vi "2_VisualizeModulePositioning.vi"(0 "Session in":T1, 1 "Calibrated positions of fiducials [mm]":dbl[][](array[numeric])=[[-675.4228165149058, -196.82430550413875, -11.55], [-579.8428201474238, -196.8506568257386, -11.55], [-579.816468825824, -101.27066045825673, -11.55], [-675.3964651933059, -101.24430913665685, -11.55], [-577.422820239396, -196.8513240176017, -11.55], [-481.84282387191405, -196.87767533920157, -11.55], [-481.8164725503142, -101.29767897171968, -11.55], [-577.396468917796, -101.2713276501198, -11.55], [-479.42282396388623, -196.87834253106465, -11.55], [-383.8428275964043, -196.90469385266454, -11.55], [-383.81647627480436, -101.32469748518264, -11.55], [-479.3964726422863, -101.29834616358275, -11.55], [-381.42282768837646, -196.90536104452758, -11.55], [-285.8428313208945, -196.93171236612747, -11.55], [-285.8164799992946, -101.35171599864559, -11.55], [-381.39647636677654, -101.3253646770457, -11.55], [-283.4228314128667, -196.93237955799054, -11.55], [-187.84283504538473, -196.95873087959043, -11.55], [-187.8164837237848, -101.37873451210854, -11.55], [-283.39648009126677, -101.35238319050865, -11.55], [-185.42283513735697, -196.9593980714535, -11.55], [-89.84283876987502, -196.98574939305337, -11.55], [-89.81648744827521, -101.40575302557149, -11.55], [-185.39648381575705, -101.3794017039716, -11.55], [-87.42283886184703, -196.98641658491644, -11.55], [8.157157505634814, -197.01276790651633, -11.55], [8.183508827234618, -101.43277153903443, -11.55], [-87.39648754024722, -101.40642021743454, -11.55], [10.57715741366269, -197.01343509837938, -11.55], [106.15715378114453, -197.0397864199793, -11.55], [106.18350510274433, -101.45979005249738, -11.55], [10.603508735262494, -101.4334387308975, -11.55], [108.57715368917252, -197.04045361184234, -11.55], [204.15715005665436, -197.06680493344223, -11.55], [204.18350137825416, -101.48680856596033, -11.55], [108.60350501077232, -101.46045724436046, -11.55], [206.57714996468223, -197.0674721253053, -11.55], [302.1571463321641, -197.09382344690516, -11.55], [302.1834976537639, -101.5138270794233, -11.55], [206.60350128628204, -101.4874757578234, -11.55], [304.57714624019206, -197.09449063876826, -11.55], [400.1571426076739, -197.12084196036813, -11.55], [400.1834939292737, -101.54084559288623, -11.55], [304.60349756179187, -101.51449427128635, -11.55], [402.5771425157018, -197.1215091522312, -11.55], [498.15713888318373, -197.1478604738311, -11.55], [498.18349020478354, -101.56786410634919, -11.55], [402.6034938373016, -101.5415127847493, -11.55], [500.5771387912116, -197.14852766569413, -11.55], [596.1571351586933, -197.17487898729405, -11.55], [596.1834864802931, -101.59488261981214, -11.55], [500.6034901128114, -101.56853129821225, -11.55]], 2 "Axis Speeds":T3={"X [mm/s]"=25.0, "Y [mm/s]"=12.5, "Z [mm/s]"=5.0}, 3 "Module fiducial marker":T5(ring)=enum."[None]", 4 "N modules":i32, 5 "error in (no error)":errorcluster, 6 "Templates path":path=path "C:/Users/Aerotech/Documents/BNL_ThermomechanicalStave", 7 "Calibration [um/pix]":dbl=0.25, 9 "Placement tolerance [um]":dbl=10.0, 10 "Current Image":refnum<vi>, 11 "Current stage position":refnum<vi>, 12 "Module Report":refnum<vi>, 13 "Moving":refnum<vi>) -> (14 "Session Out":T1, 19 "error out":errorcluster)   [LabVIEW 2016]
uses:
  <vilib>/userdefined/High Color/IMAQdx.ctl
  2_ModulePositioning/SingleModuleProgressReport.ctl
  <vilib>/vision/driver/NI_Vision_Acquisition_Software.lvlib
  <vilib>/vision/NI_Vision_Development_Module.lvlib
panel:
  out "delta Y":sgl
  out "delta X":sgl
  out "Current Position":T2
  in  "stop":bool
  out "Placement Monitor":T4(plugin-control)
  out "Fiducial Template":T4(plugin-control)
  out "Module Progress Report":T6(array[cluster])
  # "-101.244"
  # "-196.851"
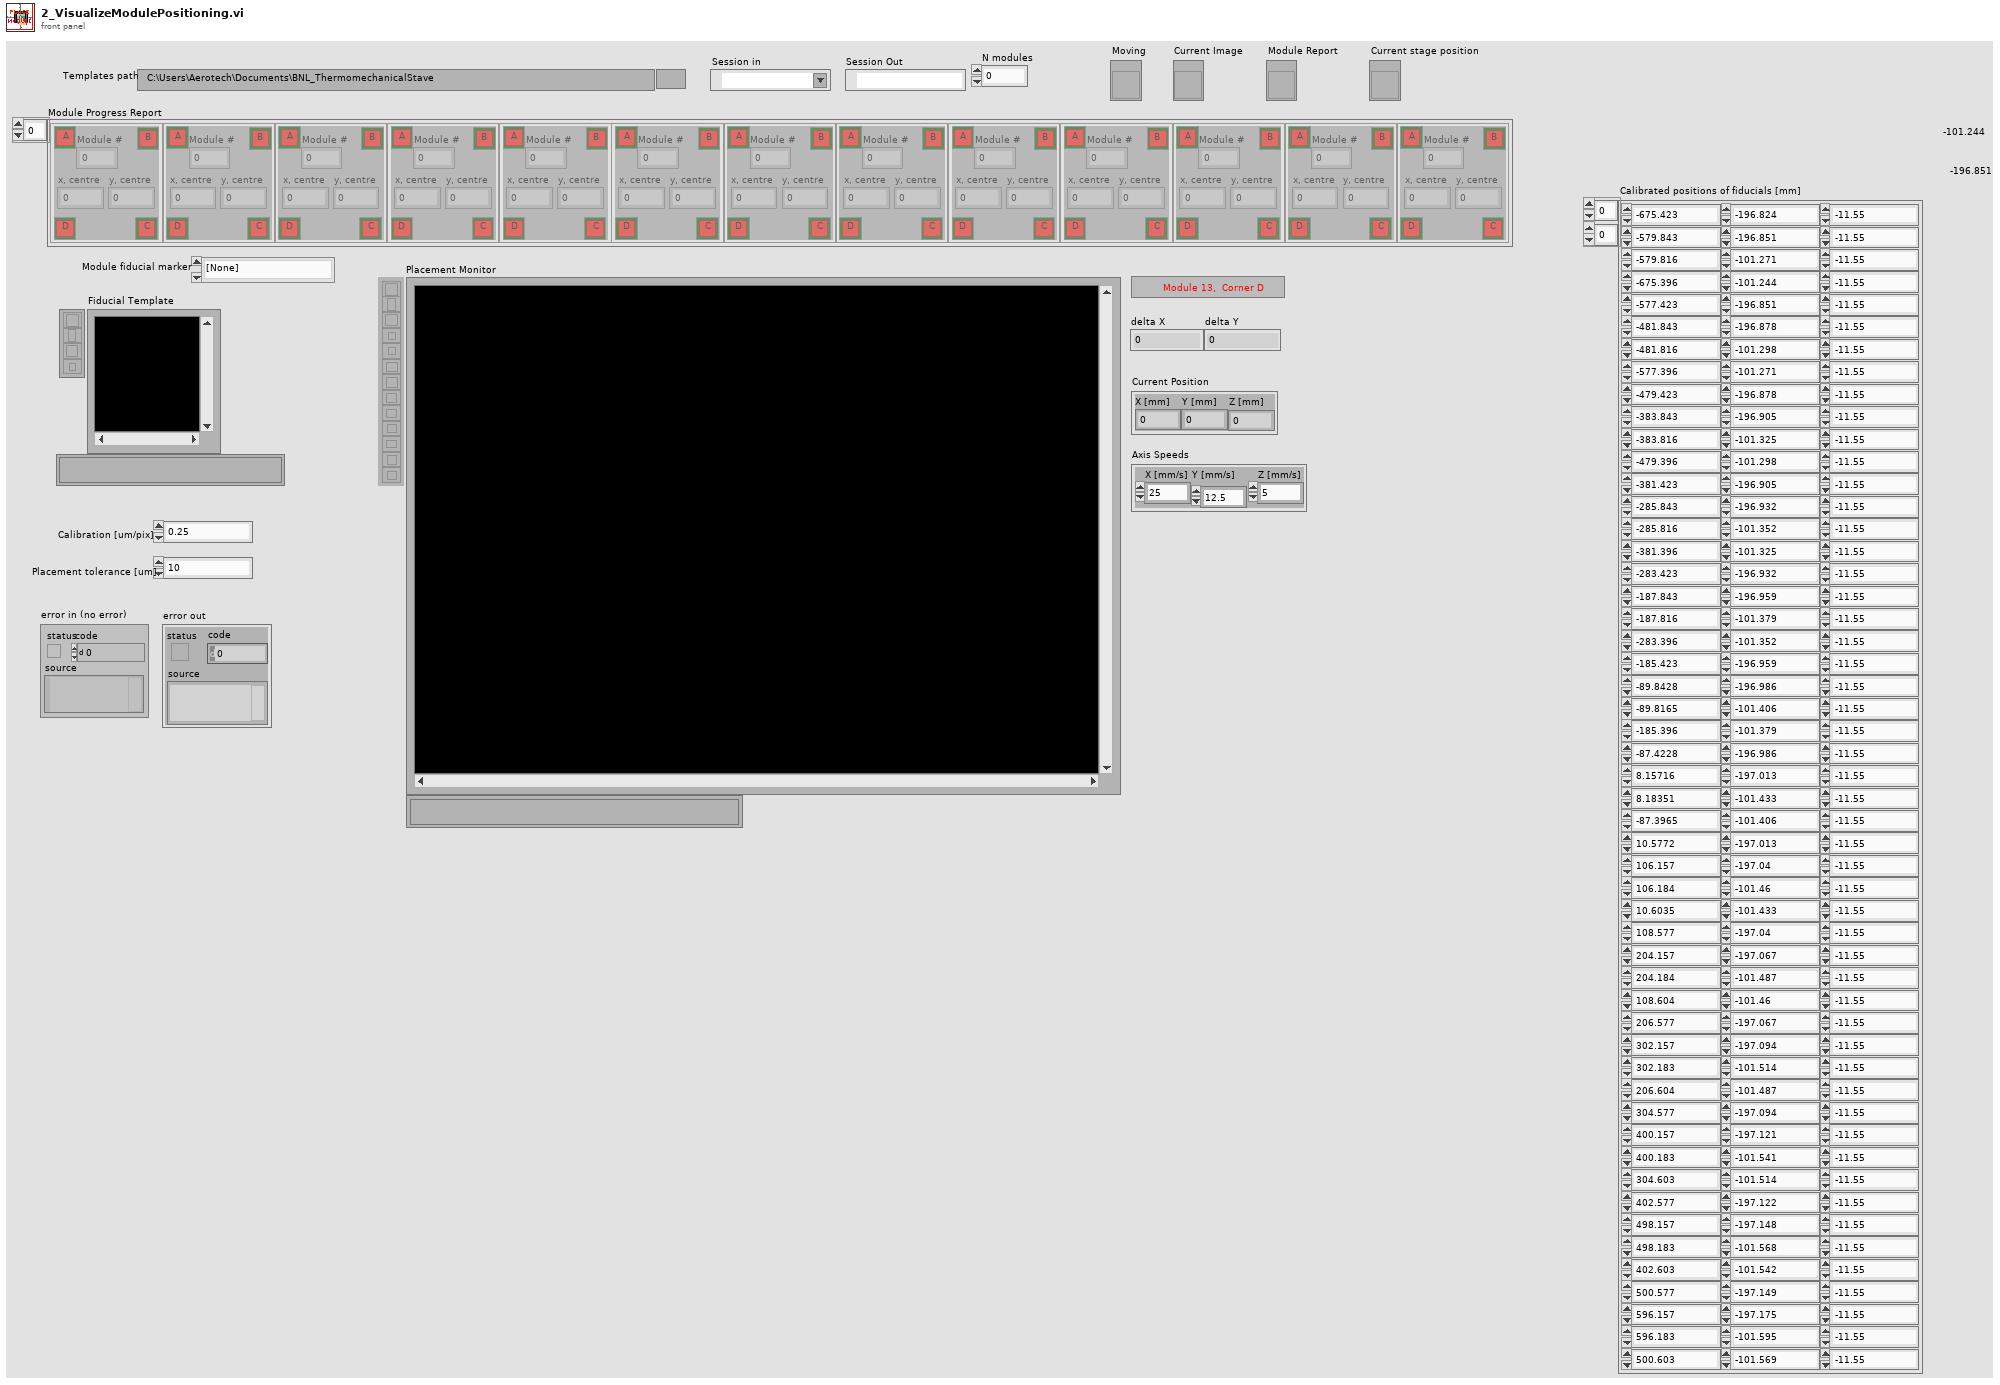
[diagram p1: front panel]
types:
  T1 = typedef "IMAQdx.ctl" = refnum<k21>
  T2 = cluster{"X [mm]":dbl, "Y [mm]":dbl, "Z [mm]":dbl}
  T3 = cluster{"X [mm/s]":dbl, "Y [mm/s]":dbl, "Z [mm/s]":dbl}
  T4 = typedef "IMAQ Image.ctl" = refnum<image>
  T5 = enum16{"Mark C", "Mark B", "Strip Corner", "[None]"}
  T6 = cluster{"A":bool, "x, centre":dbl, "y, centre":dbl, "Module #":i32, "B":bool, "D":bool, "C":bool}[]
  T7 = typedef "SingleModuleProgressReport.ctl" = cluster{"A":bool, "x, centre":dbl, "y, centre":dbl, "Module #":i32, "B":bool, "D":bool, "C":bool}
  T8 = cluster{"Algorithm":i32, "Number of Matches Requested":i32, "Minimum Match Score":sgl, "SubPixel Accuracy":bool, "Rotation Angle Ranges":cluster{"Start":sgl, "End":sgl}[], "Show Search Area":bool, "Show Result":bool}
  T9 = cluster{"Final X":dbl, "Final Y":dbl, "Final Z":dbl}
  T10 = cluster{"Position":cluster{"x":sgl, "y":sgl}, "Angle":sgl, "Scale":sgl, "Score":sgl, "Bounding Box":cluster{"x":sgl, "y":sgl}[]}[]
  T11 = cluster{"Position":cluster{"x":sgl, "y":sgl}, "Angle":sgl, "Scale":sgl, "Score":sgl, "Bounding Box":cluster{"x":sgl, "y":sgl}[]}
  T12 = cluster{"A":bool, "x, centre":dbl, "y, centre":dbl, "Module #":i32, "B":bool, "D":bool, "C":bool}
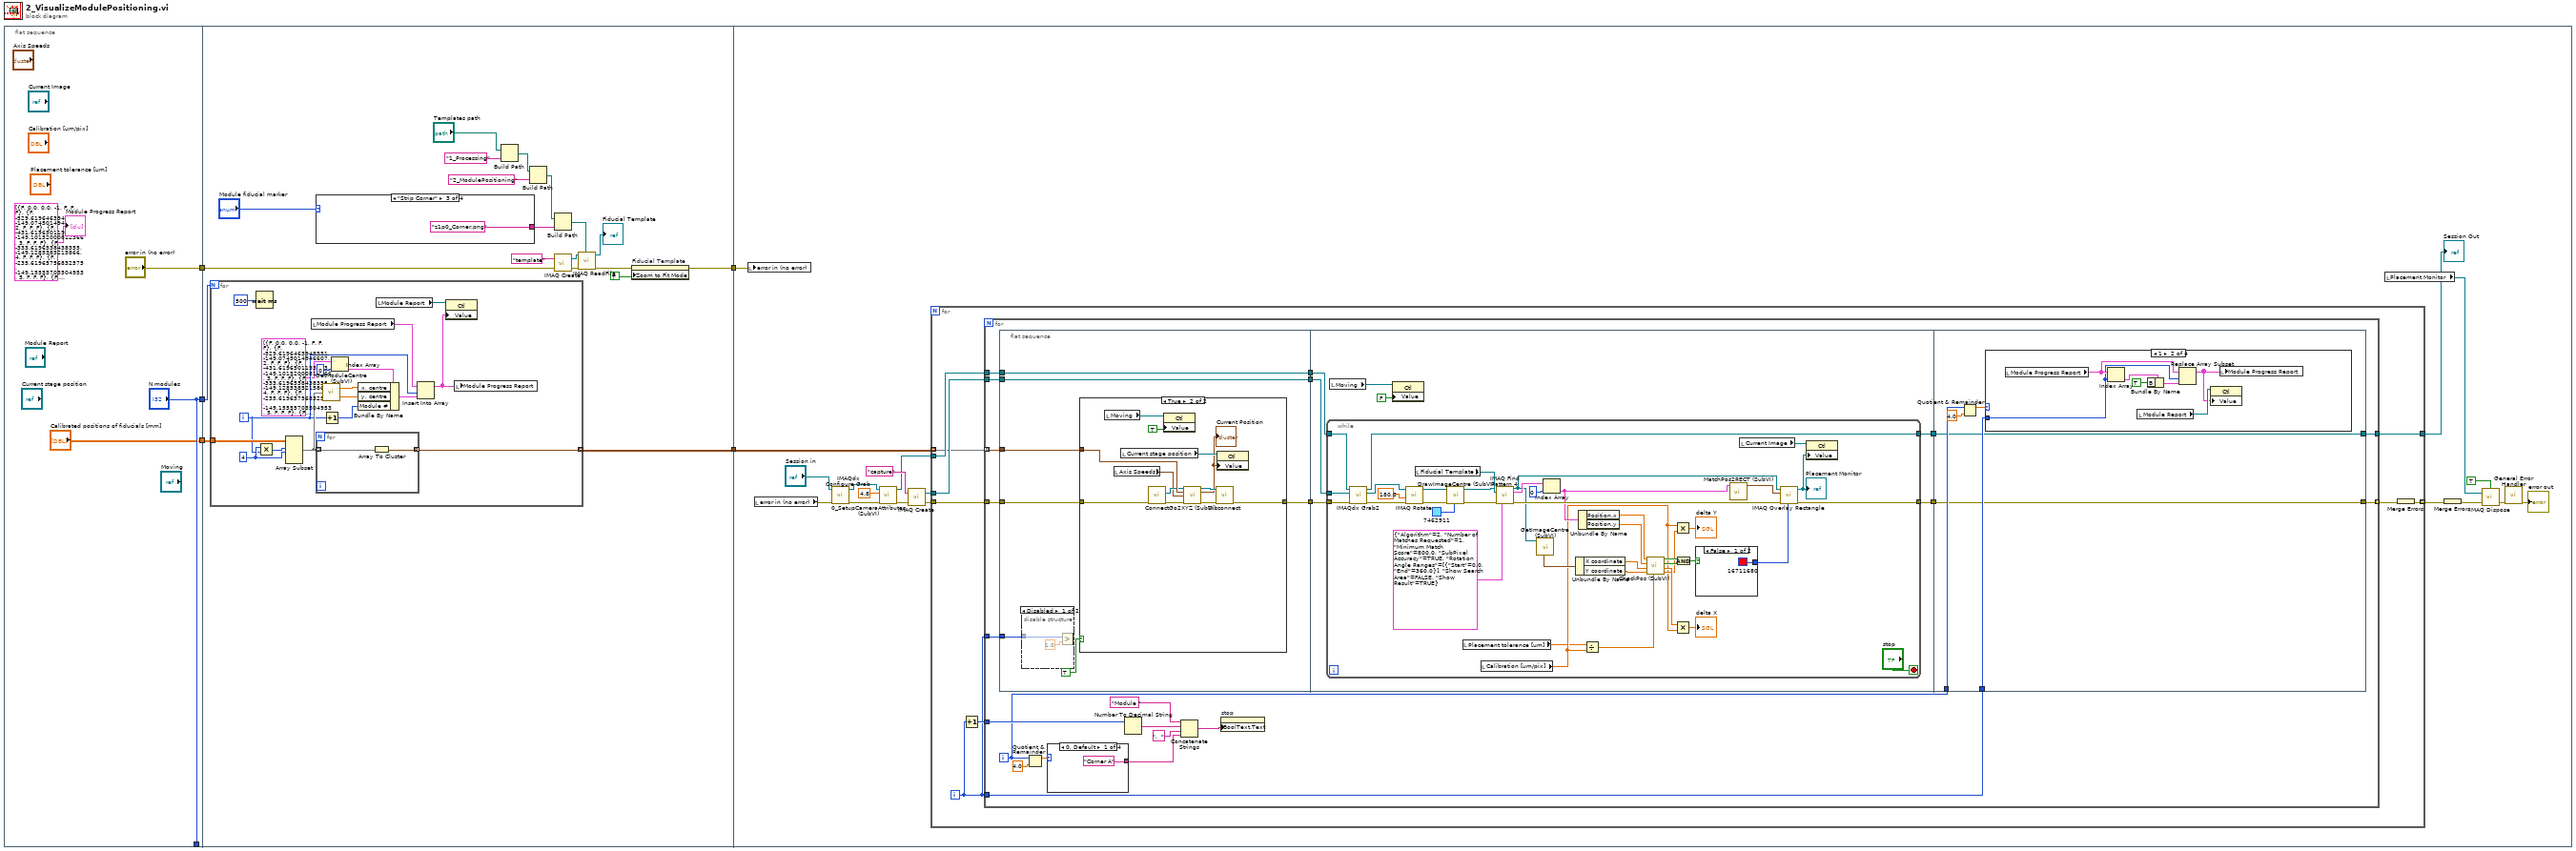
[diagram p0: block diagram]
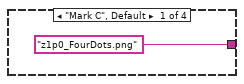
[diagram p2: hidden frame]
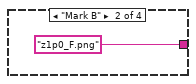
[diagram p3: hidden frame]
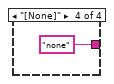
[diagram p4: hidden frame]
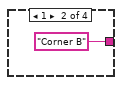
[diagram p5: hidden frame]
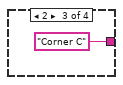
[diagram p6: hidden frame]
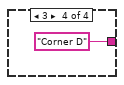
[diagram p7: hidden frame]
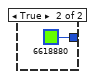
[diagram p10: hidden frame]
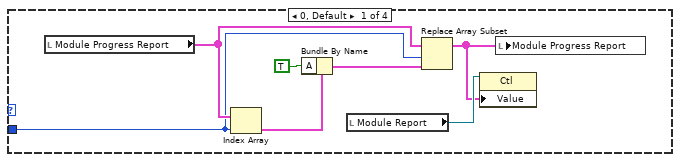
[diagram p11: hidden frame]
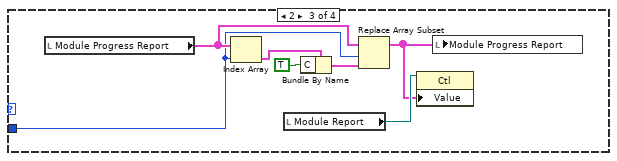
[diagram p12: hidden frame]
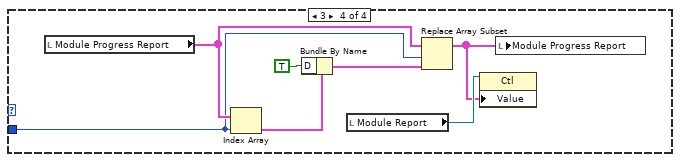
[diagram p13: hidden frame]
diagram:
  n1 = flat-sequence {
    tunnel: ["N modules"] -> _
    tunnel: ["N modules"] -> w4
    tunnel: ["Calibrated positions of fiducials [mm]"] -> w3
    tunnel: ["error in (no error)"] -> w2
    tunnel: [w26] -> w5
    tunnel: w4 -> [w28]
    tunnel: w3 -> [w27]
    tunnel: w2 -> [w11]
    tunnel: [w10] -> w1
    tunnel: w5 -> [w62]
    tunnel: w1 -> [w61]
    frame #0 {
      "Module Progress Report" <- T7[] [{"A"=FALSE, "x, centre"=0.0, "y, centre"=0.0, "Module #"=-1, "B"=FALSE, "D"=FALSE, "C"=FALSE}, {"A"=FALSE, "x, centre"=-529.6196463948551, "y, centre"=-149.0745014946607, "Module #"=2, "B"=FALSE, "D"=FALSE, "C"=FALSE}, {"A"=FALSE, "x, centre"=-431.6196501193453, "y, centre"=-149.10152000812366, "Module #"=3, "B"=FALSE, "D"=FALSE, "C"=FALSE}, {"A"=FALSE, "x, centre"=-333.6196538438355, "y, centre"=-149.1285385215866, "Module #"=4, "B"=FALSE, "D"=FALSE, "C"=FALSE}, {"A"=FALSE, "x, centre"=-235.61965756832575, "y, centre"=-149.15555703504953, "Module #"=5, "B"=FALSE, "D"=FALSE, "C"=FALSE}, {"A"=FALSE, "x, centre"=-137.6196612928161, "y, centre"=-149.1825755485125, "Module #"=6, "B"=FALSE, "D"=FALSE, "C"=FALSE}, {"A"=FALSE, "x, centre"=-627.6196426703649, "y, centre"=-149.04748298119773, "Module #"=1, "B"=FALSE, "D"=FALSE, "C"=FALSE}, {"A"=FALSE, "x, centre"=-529.6196463948551, "y, centre"=-149.0745014946607, "Module #"=2, "B"=FALSE, "D"=FALSE, "C"=FALSE}, {"A"=FALSE, "x, centre"=-431.6196501193453, "y, centre"=-149.10152000812366, "Module #"=3, "B"=FALSE, "D"=FALSE, "C"=FALSE}, {"A"=FALSE, "x, centre"=-333.6196538438355, "y, centre"=-149.1285385215866, "Module #"=4, "B"=FALSE, "D"=FALSE, "C"=FALSE}, {"A"=FALSE, "x, centre"=-235.61965756832575, "y, centre"=-149.15555703504953, "Module #"=5, "B"=FALSE, "D"=FALSE, "C"=FALSE}, {"A"=FALSE, "x, centre"=-137.6196612928161, "y, centre"=-149.1825755485125, "Module #"=6, "B"=FALSE, "D"=FALSE, "C"=FALSE}, {"A"=FALSE, "x, centre"=-39.619665017306204, "y, centre"=-149.20959406197545, "Module #"=7, "B"=FALSE, "D"=FALSE, "C"=FALSE}, {"A"=FALSE, "x, centre"=58.38033125820351, "y, centre"=-149.2366125754384, "Module #"=8, "B"=FALSE, "D"=FALSE, "C"=FALSE}, {"A"=FALSE, "x, centre"=156.38032753371334, "y, centre"=-149.26363108890132, "Module #"=9, "B"=FALSE, "D"=FALSE, "C"=FALSE}, {"A"=FALSE, "x, centre"=254.38032380922306, "y, centre"=-149.29064960236428, "Module #"=10, "B"=FALSE, "D"=FALSE, "C"=FALSE}, {"A"=FALSE, "x, centre"=352.3803200847329, "y, centre"=-149.31766811582725, "Module #"=11, "B"=FALSE, "D"=FALSE, "C"=FALSE}, {"A"=FALSE, "x, centre"=450.38031636024266, "y, centre"=-149.3446866292902, "Module #"=12, "B"=FALSE, "D"=FALSE, "C"=FALSE}, {"A"=FALSE, "x, centre"=548.3803126357524, "y, centre"=-149.37170514275314, "Module #"=13, "B"=FALSE, "D"=FALSE, "C"=FALSE}] ("Module Progress Report")
    }
    frame #1 {
      n2 = for {
        N: w28 -> [_]
        tunnel: w27 -> [w49]
        tunnel: [w46] -> w26 mode=indexing
        i -> [w37]
        w47 = 4 ("x")
        n3 = Wait (ms)(milliseconds to wait=u32 500) -> ()  [unwired: 1 out]
        n4 = Multiply(x=w47, y=w37) -> (x*y=w48:i32)
        n5 = Array Subset(array=w49, index (row)=w48, length (row)=w47) -> (w45:dbl[][])  [unwired: 2 in]
        n6 = local read "Module Progress Report"() -> (w38:T6)
        n7 = for {
          tunnel: w45 -> [w50] mode=indexing
          tunnel: [w51] -> w46 mode=indexing
          n8 = Array To Cluster(array=w50) -> (cluster=w51:cluster{"[0]":dbl, "[1]":dbl, "[2]":dbl})
        }
        n9 = call "GetModuleCentre (SubVI).vi"("4x3 Array of Fiducial Coordinates"=w45) -> ("x, centre"=w44:dbl, "y, centre"=w43:dbl)
        n10 = Increment(x=w37) -> (x+1=w42:i32)
        n11 = Index Array(array=T7[] [{"A"=FALSE, "x, centre"=0.0, "y, centre"=0.0, "Module #"=-1, "B"=FALSE, "D"=FALSE, "C"=FALSE}, {"A"=FALSE, "x, centre"=-529.6196463948551, "y, centre"=-149.0745014946607, "Module #"=2, "B"=FALSE, "D"=FALSE, "C"=FALSE}, {"A"=FALSE, "x, centre"=-431.6196501193453, "y, centre"=-149.10152000812366, "Module #"=3, "B"=FALSE, "D"=FALSE, "C"=FALSE}, {"A"=FALSE, "x, centre"=-333.6196538438355, "y, centre"=-149.1285385215866, "Module #"=4, "B"=FALSE, "D"=FALSE, "C"=FALSE}, {"A"=FALSE, "x, centre"=-235.61965756832575, "y, centre"=-149.15555703504953, "Module #"=5, "B"=FALSE, "D"=FALSE, "C"=FALSE}, {"A"=FALSE, "x, centre"=-137.6196612928161, "y, centre"=-149.1825755485125, "Module #"=6, "B"=FALSE, "D"=FALSE, "C"=FALSE}, {"A"=FALSE, "x, centre"=-627.6196426703649, "y, centre"=-149.04748298119773, "Module #"=1, "B"=FALSE, "D"=FALSE, "C"=FALSE}, {"A"=FALSE, "x, centre"=-529.6196463948551, "y, centre"=-149.0745014946607, "Module #"=2, "B"=FALSE, "D"=FALSE, "C"=FALSE}, {"A"=FALSE, "x, centre"=-431.6196501193453, "y, centre"=-149.10152000812366, "Module #"=3, "B"=FALSE, "D"=FALSE, "C"=FALSE}, {"A"=FALSE, "x, centre"=-333.6196538438355, "y, centre"=-149.1285385215866, "Module #"=4, "B"=FALSE, "D"=FALSE, "C"=FALSE}, {"A"=FALSE, "x, centre"=-235.61965756832575, "y, centre"=-149.15555703504953, "Module #"=5, "B"=FALSE, "D"=FALSE, "C"=FALSE}, {"A"=FALSE, "x, centre"=-137.6196612928161, "y, centre"=-149.1825755485125, "Module #"=6, "B"=FALSE, "D"=FALSE, "C"=FALSE}, {"A"=FALSE, "x, centre"=-39.619665017306204, "y, centre"=-149.20959406197545, "Module #"=7, "B"=FALSE, "D"=FALSE, "C"=FALSE}, {"A"=FALSE, "x, centre"=58.38033125820351, "y, centre"=-149.2366125754384, "Module #"=8, "B"=FALSE, "D"=FALSE, "C"=FALSE}, {"A"=FALSE, "x, centre"=156.38032753371334, "y, centre"=-149.26363108890132, "Module #"=9, "B"=FALSE, "D"=FALSE, "C"=FALSE}, {"A"=FALSE, "x, centre"=254.38032380922306, "y, centre"=-149.29064960236428, "Module #"=10, "B"=FALSE, "D"=FALSE, "C"=FALSE}, {"A"=FALSE, "x, centre"=352.3803200847329, "y, centre"=-149.31766811582725, "Module #"=11, "B"=FALSE, "D"=FALSE, "C"=FALSE}, {"A"=FALSE, "x, centre"=450.38031636024266, "y, centre"=-149.3446866292902, "Module #"=12, "B"=FALSE, "D"=FALSE, "C"=FALSE}, {"A"=FALSE, "x, centre"=548.3803126357524, "y, centre"=-149.37170514275314, "Module #"=13, "B"=FALSE, "D"=FALSE, "C"=FALSE}] ("Module Progress Report"), index=0) -> (element=w39:T7)
        n12 = Bundle By Name(cluster=w39, "x, centre"=w44, "y, centre"=w43, "Module #"=w42) -> (w35:T7)
        n13 = local read "Module Report"() -> (w34:refnum<vi>)
        n14 = Insert Into Array(array=w38, index=w37, new element=w35) -> (w33:T6)
        n15 = property class="Ctl"(reference=w34, "Value"=w33) -> ()  [unwired: 1 in, 2 out]
        n16 = local write "Module Progress Report"(w33) -> ()
      }
      n17 = case shown="\"Strip Corner\"" "Module fiducial marker" {
        tunnel: ["z1p0_FourDots.png" ("name or relative path") "z1p0_F.png" ("name or relative path") "z1p0_Corner.png" ("name or relative path") "none" ("name or relative path")] -> w25
        frame "Mark C", Default {
        }
        frame "Mark B" {
        }
        frame "Strip Corner" {
        }
        frame "[None]" {
        }
      }
      n18 = Build Path(base path="Templates path", name or relative path="1_Processing") -> (appended path=w12:path)
      n19 = Build Path(base path=w12, name or relative path="2_ModulePositioning") -> (appended path=w23:path)
      n20 = Build Path(base path=w23, name or relative path=w25) -> (appended path=w22:path)
      n21 = call "IMAQ Create"("Image Name"="template", "error in (no error)"=w11) -> ("New Image"=w21:T4, "error out"=w20:errorcluster)  [unwired: 3 in]
      n22 = call "IMAQ ReadFile"("File Path"=w22, "error in (no error)"=w20, "Image"=w21) -> ("error out"=w16:errorcluster, "Image Out"=→"Fiducial Template":T4)  [unwired: 4 in, 3 out]
      n23 = property on="Fiducial Template" class="ImageControl"(error in=w16, "Zoom to Fit Mode"=TRUE) -> (error out=w10:errorcluster)  [unwired: 1 in, 1 out]
    }
    frame #2 {
      n24 = local write "error in (no error)"(w61) -> ()
      n25 = local read "error in (no error)"() -> (w60:errorcluster)
      n26 = call <vilib>:"IMAQdx Configure Grab.vi"("error in"=w60, "Session In"="Session in") -> ("error out"=w69:errorcluster, "Session Out"=w70:T1)  [unwired: 8 out]
      n27 = call "0_SetupCameraAttributes (SubVI).vi"("error in (no error)"=w69, "Gain"=4.8, "Camera session in"=w70) -> ("error out"=w67:errorcluster, "Camera session out"=w64:T1)  [unwired: 7 in]
      n28 = call "IMAQ Create"("Image Name"="capture", "error in (no error)"=w67) -> ("New Image"=w65:T4, "error out"=w63:errorcluster)  [unwired: 3 in]
      n29 = for {
        tunnel: w64 -> [w79]
        tunnel: w65 -> [w78]
        tunnel: w63 -> [w77]
        tunnel: w62 -> [w75] mode=indexing
        tunnel: [w72] -> w59 mode=indexing
        tunnel: [w71] -> w57
        i -> [w74]
        n30 = Increment(x=w74) -> (x+1=w76:i32)
        n31 = for {
          tunnel: w79 -> [w98]
          tunnel: w78 -> [w97]
          tunnel: w77 -> [w96]
          tunnel: w76 -> [w91]
          tunnel: w75 -> [w87] mode=indexing
          tunnel: w74 -> [w86]
          tunnel: w74 -> [w84]
          tunnel: [w82] -> w73 mode=indexing
          tunnel: [w80] -> w71
          i -> [w85]
          n32 = flat-sequence {
            tunnel: w98 -> [w111]
            tunnel: w96 -> [w110]
            tunnel: w97 -> [w112]
            tunnel: [w112] -> w101
            tunnel: [w109] -> w100
            tunnel: [w111] -> w99
            tunnel: w87 -> [w108]
            tunnel: w84 -> [w107]
            tunnel: w101 -> [w134]
            tunnel: w100 -> [w133]
            tunnel: w99 -> [w132]
            tunnel: [w131] -> w83
            tunnel: [w130] -> w81
            tunnel: w86 -> [w180]
            tunnel: w85 -> [w179]
            tunnel: w83 -> [w178]
            tunnel: [w178] -> w82
            tunnel: [w177] -> w80
            tunnel: w81 -> [w177]
            frame #0 {
              n33 = disable-structure shown="Disabled" {
                disable-tunnel: w107 -> [w114 _]
                frame Disabled {
                  n34 = Greater?(x=w114, y=1.0) -> ()  [unwired: 1 out]
                }
                frame Enabled {
                }
              }
              n35 = case shown="True" TRUE {
                tunnel: w110 -> [w115 w127]
                tunnel: [w115 w126] -> w109
                tunnel: w108 -> [_ w125]
                frame False {
                  # "Temporarily skip corners C and D"
                }
                frame True {
                  n36 = local read "Moving"() -> (w117:refnum<vi>)
                  n37 = local read "Axis Speeds"() -> (w120:T3)
                  n38 = local read "Current stage position"() -> (w119:refnum<vi>)
                  n39 = call "Connect.vi"("error in (no error)"=w127) -> ("error out"=w124:errorcluster, "controller"=w123:refnum<k24>)  [unwired: 9 in]
                  n40 = property class="Ctl"(reference=w117, "Value"=TRUE) -> ()  [unwired: 1 in, 2 out]
                  n41 = call "Go2XYZ (SubVI).vi"(".NET Refnum in"=w123, "Go to Coordinates"=w125, "Axis Speeds"=w120, "error in (no error)"=w124) -> (".NET Refnum out"=w122:refnum<k24>, "Final Position"=w118:T9, "error out"=w121:errorcluster)  [unwired: 7 in, 2 out]
                  "Current Position" <- w118
                  n42 = call "Disconnect.vi"("error in (no error)"=w121, "controller"=w122) -> ("error out"=w126:errorcluster)  [unwired: 9 in]
                  n43 = property class="Ctl"(reference=w119, "Value"=w118) -> ()  [unwired: 1 in, 2 out]
                }
              }
            }
            frame #1 {
              n44 = while {
                tunnel: w134 -> [w174]
                tunnel: w133 -> [w173]
                tunnel: w132 -> [w172]
                tunnel: [w168] -> w130
                tunnel: [w160] -> w131
                stop <- "stop" stop-if-true
                n45 = call <vilib>:"IMAQdx Grab2.vi"("error in"=w173, "Image In"=w174, "Session In"=w172) -> ("error out"=w169:errorcluster, "Image Out"=w171:T4, "Session Out"=w168:T1)  [unwired: 5 in, 1 out]
                n46 = call "IMAQ Rotate"("error in (no error)"=w169, "Angle (degrees)"=sgl 180.0, "Image Src"=w171) -> ("error out"=w142:errorcluster, "Image Dst Out"=w144:T4)  [unwired: 7 in]
                n47 = local read "Fiducial Template"() -> (w165:T4)
                n48 = call "DrawImageCentre (SubVI).vi"("Axis colour"=u32 7462911, "error in (no error)"=w142, "Refnum in"=w144) -> ("error out"=w141:errorcluster, "Refnum out"=w143:T4)  [unwired: 7 in]
                n49 = local read "Placement tolerance [um]"() -> (w137:dbl)
                n50 = local read "Calibration [um/pix]"() -> (w138:dbl)
                n51 = call "IMAQ Find Pattern 4"("Image"=w143, "Template"=w165, "error in"=w141, "Settings"=T8 {"Algorithm"=2, "Number of Matches Requested"=1, "Minimum Match Score"=800.0, "SubPixel Accuracy"=TRUE, "Rotation Angle Ranges"=[{"Start"=0.0, "End"=360.0}], "Show Search Area"=FALSE, "Show Result"=TRUE}) -> ("Image Out"=w155:T4, "Matches (pixel)"=w163:T10, "error out"=w161:errorcluster)  [unwired: 5 in, 4 out]
                n52 = call "GetImageCentre (SubVI).vi"("Image in \n(refnum)"=w155) -> ("Centre Point"=w154:cluster{"X coordinate":dbl, "Y coordinate":dbl})  [unwired: 4 in, 4 out]
                n53 = Index Array(array=w163, index=0) -> (element=w149:T11)
                n54 = Unbundle By Name(w154) -> ("X coordinate"=w153:dbl, "Y coordinate"=w152:dbl)
                n55 = Unbundle By Name(w149) -> ("Position.x"=w159:sgl, "Position.y"=w158:sgl)
                n56 = Divide(x=w137, y=w138) -> (x/y=w139:dbl)
                n57 = call "CheckPos (SubVI).vi"("x"=w159, "y"=w158, "true x"=w153, "true y"=w152, "variation tolerance"=w139) -> ("pass x coordinate"=w157:bool, "pass y coordinate"=w156:bool, "delta X"=w148:sgl, "delta Y"=w147:sgl)  [unwired: 2 in]
                n58 = Multiply(x=w138, y=w147) -> (x*y=→"delta Y":dbl)
                n59 = Multiply(x=w148, y=w138) -> (x*y=→"delta X":dbl)
                n60 = And(x=w157, y=w156) -> (x .and. y?=w151:bool)
                n61 = case shown="False" w151 {
                  tunnel: [u32 16711680 ("Color") u32 6618880 ("Color")] -> w150
                  frame False {
                  }
                  frame True {
                  }
                }
                n62 = call "MatchPos2RECT (SubVI).vi"("Match element"=w149) -> ("Rectangle"=w164:cluster{"x":sgl, "y":sgl, dbl, dbl})  [unwired: 10 in]
                n63 = local read "Current Image"() -> (w136:refnum<vi>)
                n64 = call "IMAQ Overlay Rectangle"("Color"=w150, "error in (no error)"=w161, "Rectangle"=w164, "Image"=w155) -> ("error out"=w160:errorcluster, "Image Out"=w135:T4)  [unwired: 6 in]
                "Placement Monitor" <- w135
                n65 = property class="Ctl"(reference=w136, "Value"=w135) -> ()  [unwired: 1 in, 2 out]
              }
              n66 = local read "Moving"() -> (w128:refnum<vi>)
              n67 = property class="Ctl"(reference=w128, "Value"=FALSE) -> ()  [unwired: 1 in, 2 out]
            }
            frame #2 {
              n68 = Quotient & Remainder(x=w179, y=4.0) -> (x-y*floor(x/y)=w182:dbl)  [unwired: 1 out]
              n69 = case shown="1" w182 {
                tunnel: w180 -> [w186 w192 w199 w206]
                frame 0, Default {
                  n70 = local read "Module Progress Report"() -> (w187:T6)
                  n71 = Index Array(array=w187, index=w186) -> (element=w185:T12)
                  n72 = Bundle By Name(cluster=w185, "A"=TRUE) -> (w188:T12)
                  n73 = local read "Module Report"() -> (w184:refnum<vi>)
                  n74 = Replace Array Subset(array=w187, new element=w188, index=w186) -> (w183:T6)
                  n75 = property class="Ctl"(reference=w184, "Value"=w183) -> ()  [unwired: 1 in, 2 out]
                  n76 = local write "Module Progress Report"(w183) -> ()
                }
                frame 1 {
                  n77 = local read "Module Progress Report"() -> (w194:T6)
                  n78 = Index Array(array=w194, index=w192) -> (element=w193:T12)
                  n79 = local read "Module Report"() -> (w191:refnum<vi>)
                  n80 = Bundle By Name(cluster=w193, "B"=TRUE ("A")) -> (w195:T12)
                  n81 = Replace Array Subset(array=w194, new element=w195, index=w192) -> (w190:T6)
                  n82 = property class="Ctl"(reference=w191, "Value"=w190) -> ()  [unwired: 1 in, 2 out]
                  n83 = local write "Module Progress Report"(w190) -> ()
                }
                frame 2 {
                  n84 = local read "Module Progress Report"() -> (w201:T6)
                  n85 = Index Array(array=w201, index=w199) -> (element=w200:T12)
                  n86 = local read "Module Report"() -> (w198:refnum<vi>)
                  n87 = Bundle By Name(cluster=w200, "C"=TRUE ("A")) -> (w202:T12)
                  n88 = Replace Array Subset(array=w201, new element=w202, index=w199) -> (w197:T6)
                  n89 = property class="Ctl"(reference=w198, "Value"=w197) -> ()  [unwired: 1 in, 2 out]
                  n90 = local write "Module Progress Report"(w197) -> ()
                }
                frame 3 {
                  n91 = local read "Module Progress Report"() -> (w208:T6)
                  n92 = Index Array(array=w208, index=w206) -> (element=w207:T12)
                  n93 = Bundle By Name(cluster=w207, "D"=TRUE ("A")) -> (w209:T12)
                  n94 = local read "Module Report"() -> (w205:refnum<vi>)
                  n95 = Replace Array Subset(array=w208, new element=w209, index=w206) -> (w204:T6)
                  n96 = property class="Ctl"(reference=w205, "Value"=w204) -> ()  [unwired: 1 in, 2 out]
                  n97 = local write "Module Progress Report"(w204) -> ()
                }
              }
            }
          }
          n98 = Quotient & Remainder(x=w85, y=4.0) -> (x-y*floor(x/y)=w88:dbl)  [unwired: 1 out]
          n99 = case shown="0, Default" w88 {
            tunnel: ["Corner A" "Corner B" "Corner C" "Corner D"] -> w90
            frame 0, Default {
            }
            frame 1 {
            }
            frame 2 {
            }
            frame 3 {
            }
          }
          n100 = Number To Decimal String(number=w91) -> (decimal integer string=w94:string)  [unwired: 1 in]
          n101 = Concatenate Strings("Module " ("string"), w94, ",  " ("string"), w90) -> (w95:string)
          n102 = property on="stop" class="Bool"("BoolText.Text"=w95) -> ()  [unwired: 2 in, 2 out]
        }
        n103 = Merge Errors(w73) -> (w72:errorcluster)
      }
      "Session Out" <- w57
      n104 = local read "Placement Monitor"() -> (w55:T4)
      n105 = Merge Errors(w59) -> (w52:errorcluster)
      n106 = call "IMAQ Dispose"("All Images? (No)"=TRUE, "Image"=w55, "error in (no error)"=w52) -> ("error out"=w53:errorcluster)  [unwired: 3 in]
      n107 = call <vilib>:"General Error Handler.vi"("error in (no error)"=w53) -> ("error out"=→"error out":errorcluster)  [unwired: 10 in, 4 out]
    }
  }
